vi "Create Wheel Angular Velocity Row.vi"(8 "error in (no error)":errorcluster, 10 "steering angle (rad)":dbl, 11 "fixed wheel in":refnum<class "NI_Robotics_Fixed Wheel.lvclass">) -> (0 "error out":errorcluster, 2 "wheel angular velocity row":dbl[](array[numeric]), 3 "fixed wheel out":refnum<class "NI_Robotics_Fixed Wheel.lvclass">)   [LabVIEW 2017, in "NI_Robotics_Fixed Wheel.lvclass"]
uses:
  <vilib>/robotics/Steering/Fixed Wheel/NI_Robotics_Fixed Wheel.lvclass
  c:/Program Files (x86)/National Instruments/LabVIEW 2017/vi.lib/robotics/Steering/Wheel/NI_Robotics_Wheel.lvclass
  <vilib>/robotics/Steering/Wheel/NI_Robotics_Wheel.lvclass/NI_Robotics_Wheel.ctl
  <vilib>/robotics/Steering/Wheel/NI_Robotics_Wheel.lvclass
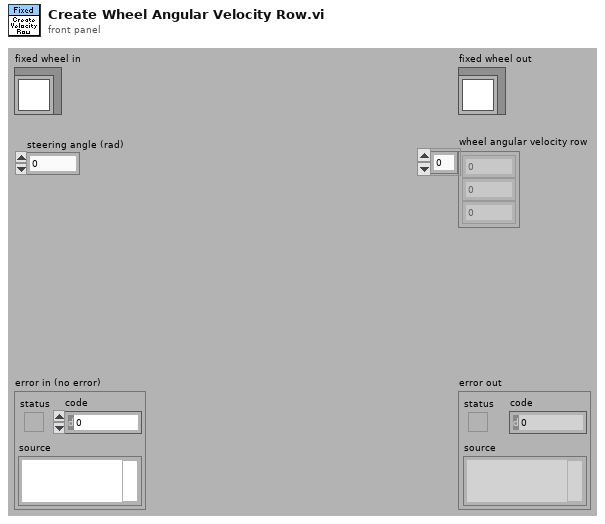
[diagram p1: front panel]
types:
  T1 = typedef "NI_Matrix.lvlib/RealMatrix.ctl" = dbl[][]
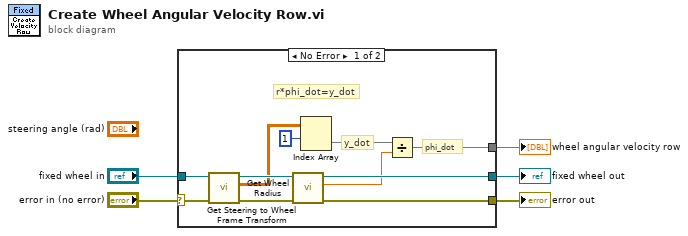
[diagram p0: block diagram]
diagram:
  n1 = case shown="No Error" "error in (no error)" {
    selector: "error in (no error)" -> [w8 w18]
    tunnel: [w15 w18] -> w4
    tunnel: "fixed wheel in" -> [w10 w17]
    tunnel: [w16 w17] -> w2
    tunnel: [w13 _] -> w1
    frame No Error {
      # "phi_dot"
      # "y_dot"
      # "r*phi_dot=y_dot"
      n2 = call <vilib>:"Get Steering to Wheel Frame Transform.vi"("error in (no error)"=w8, "wheel in"=w10) -> ("error out"=w7:errorcluster, "steering to wheel frame transform"=w6:T1, "wheel out"=w9:refnum<class "NI_Robotics_Fixed Wheel.lvclass">)  [unwired: 7 in]
      n3 = call <vilib>:"Get Wheel Radius.vi"("error in (no error)"=w7, "wheel in"=w9) -> ("error out"=w15:errorcluster, "wheel radius"=w14:dbl, "wheel out"=w16:refnum<class "NI_Robotics_Fixed Wheel.lvclass">)  [unwired: 7 in]
      n4 = Index Array(array=w6, index (row)=1) -> (element=w11:dbl[])  [unwired: 1 in]
      n5 = Divide(x=w11, y=w14) -> (x/y=w13:dbl[])
    }
    frame Error {
    }
  }
  "error out" <- w4
  "fixed wheel out" <- w2
  "wheel angular velocity row" <- w1
